vi "Write To Spreadsheet File2.vi"(0 "delimiter (Tab)":string="\t", 1 "transpose? (no:F)":bool, 2 "dialogue":string="Choose file to write", 4 "format (%.3f)":string="%.3f", 5 "append to file? (new file:F)":bool, 6 "1D data":sgl[](array[numeric]) format="%.2f", 7 "2D data":sgl[][](array[numeric]) format="%.2f", 8 "file path (dialog if empty)":path) -> (3 "new file path (Not A Path if cancelled)":path)   [LabVIEW 2018]
doc: "Converts a 2D or 1D array of single-precision numbers to a text string and writes the string to a new byte stream file or appends the string to an existing file. You can optionally transpose the data. This VI opens or creates the file beforehand and closes it afterwards. You can use this VI to create a text file readable by most spreadsheet applications.\n\nfile path is the path name of the file. If file path is empty (default value) or is Not A Path, the VI displays a File dialog box from which you can select a file. Error 43 occurs if the user cancels the dialog. \n\n2D data contains the single-precision numbers the VI writes to the file if 1D data is not wired or is empty.\n\n1D data contains the single-precision numbers the VI writes to the file if this input is not empty. The VI converts the 1D array into a 2D array before transposing it and converting it to a string and writing it to the file. If transpose? is FALSE, each call to this VI creates a new line or row in the file.\n\nappend to file? Set to TRUE if you want to append the data to a existing file; you can also set it TRUE to write to a new file. Set to FALSE (default value) if you want to write the data to a new file or to replace an existing file. \n\ntranspose? Set TRUE to transpose the data before converting it to a string. The default value is FALSE.\n\nformat specifies how to convert the numbers to characters. If the format string is %.3f (default), the VI creates a string long enough to contain the number, with three digits to the right of the decimal point. If the format is %d, the VI converts the data to integer form using as many characters as necessary to contain the entire number. Refer to the discussion of format strings and the Array To Spreadsheet String function in Chapter 6, String Functions, of the LabVIEW Function Reference Manual.\n\nnew file path is the path of the file to which the VI wrote data. You can use this output to determine the path of a file that you open using dialog. new file path returns Not A Path if the user selects Cancel from the dialog box."
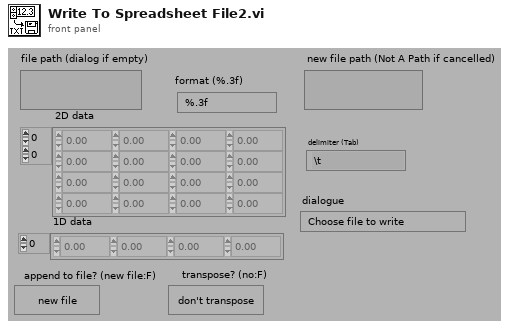
[diagram p1: front panel]
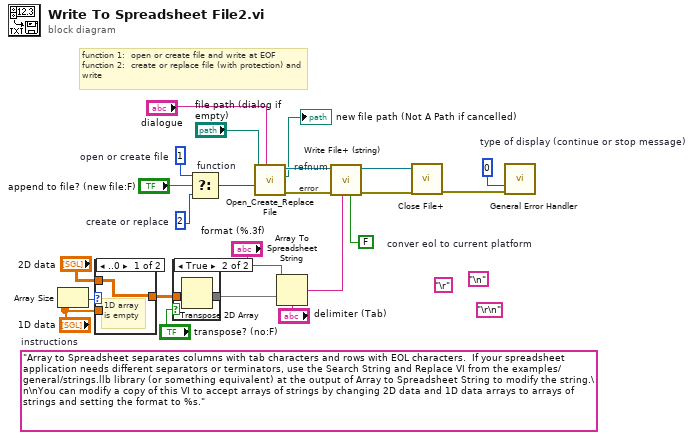
[diagram p0: block diagram]
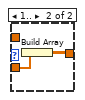
[diagram p3: hidden frame]
diagram:
  (unwired) "\r\n"
  (unwired) "\n"
  (unwired) "\r"
  (unwired) "Array to Spreadsheet separates columns with tab characters and rows with EOL characters.  If your spreadsheet application needs different separators or terminators, use the Search String and Replace VI from the examples/general/strings.llb library (or something equivalent) at the output of Array to Spreadsheet String to modify the string.\n\nYou can modify a copy of this VI to accept arrays of strings by changing 2D data and 1D data arrays to arrays of strings and setting the format to %s."  # instructions
  w4 = i16 2  # create or replace
  w7 = FALSE  # conver eol to current platform
  w21 = 0  # type of display (continue or stop message)
  w22 = i16 1  # open or create file
  # "error"
  # "refnum"
  # "function 1:  open or create file and write at EOF\nfunction 2:  create or replace file (with protection) and write"
  n1 = Array Size(array="1D data") -> (size(s)=w19:i32)
  n2 = case shown="..0" w19 {
    tunnel: "1D data" -> [_ w26]
    tunnel: [w24 w25] -> w15
    tunnel: "2D data" -> [w24 _]
    frame ..0 {
      # "1D array is empty"
    }
    frame 1.. {
      n3 = Build Array(w26) -> (w25:sgl[][])
    }
  }
  n4 = case shown="True" "transpose? (no:F)" {
    tunnel: [w27 w29] -> w13
    tunnel: w15 -> [w27 w28]
    frame False {
    }
    frame True {
      n5 = Transpose 2D Array(2D array=w28) -> (transposed array=w29:sgl[][])
    }
  }
  n6 = Select "function"(t=w22, s="append to file? (new file:F)", f=w4) -> (s? t:f=w12:i16)
  n7 = call <vilib>:"Open_Create_Replace File.vi"("prompt"="dialogue", "function (open:0)"=w12, "file path"="file path (dialog if empty)") -> ("error out"=w10:errorcluster, "new file path"=→"new file path (Not A Path if cancelled)":path, "refnum"=w6:refnum<file>)  [unwired: 5 in, 1 out]
  n8 = Array To Spreadsheet String(delimiter (Tab)="delimiter (Tab)", array=w13, 3:"format (%.3f)") -> (spreadsheet string=w1:string)
  n9 = call <vilib>:"Write File+ (string).vi"("convert eol? (no:F)"=w7, "string"=w1, "error in (no error)"=w10, "refnum"=w6) -> ("error out"=w20:errorcluster, "dup refnum"=w9:refnum<file>)  [unwired: 3 in, 1 out]
  n10 = call <vilib>:"Close File+.vi"("error in (no error)"=w20, "refnum"=w9) -> ("error out"=w8:errorcluster)  [unwired: 3 in, 2 out]
  n11 = call <vilib>:"General Error Handler.vi"("type of dialog (OK msg:1)"=w21, "error in (no error)"=w8) -> ()  [unwired: 9 in, 5 out]
